vi "Write Log File Directory.vi"(8 "error in (no error)":errorcluster, 10 "Log File Directory":string, 11 "Check Size Message in":refnum<class "Check Size Message.lvclass">) -> (0 "error out":errorcluster, 3 "Check Size Message out":refnum<class "Check Size Message.lvclass">)   [LabVIEW 2020, in "AIM ARINC 664 Engine.lvlib" / "Implementation.lvlib" / "Frame Logging.lvlib" / "Check Size Message.lvclass"]
uses:
  Check Size Message.lvclass
  Check Size Message.lvclass/Check Size Message.ctl
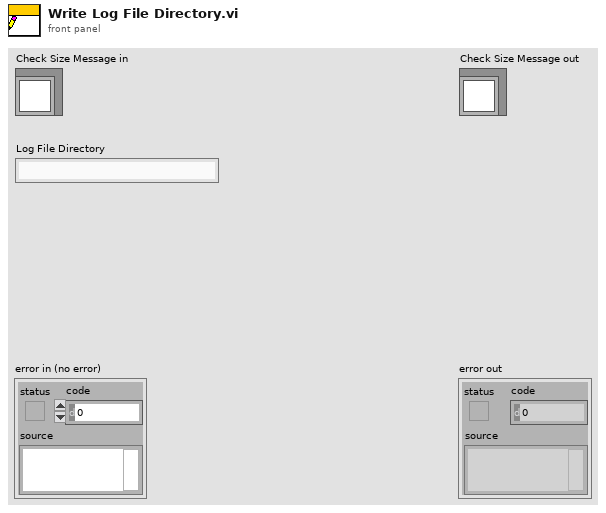
[diagram p1: front panel]
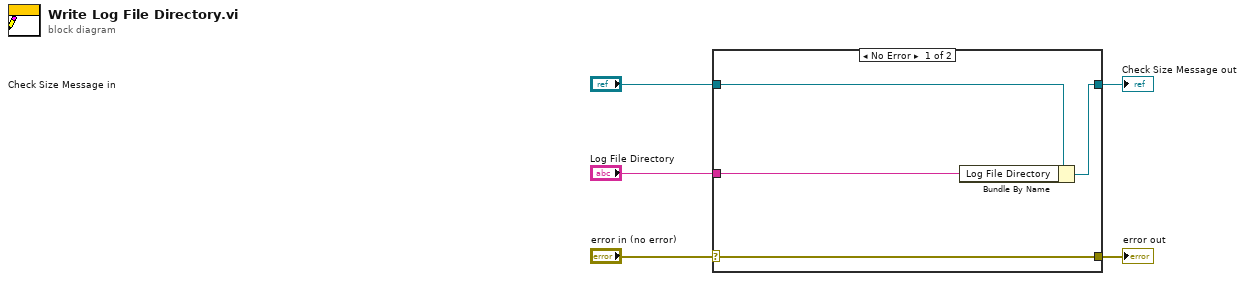
[diagram p0: block diagram]
diagram:
  n1 = case shown="No Error" "error in (no error)" {
    selector: "error in (no error)" -> [w9 w10]
    tunnel: [w9 w10] -> w4
    tunnel: [w7 w11] -> w2
    tunnel: "Check Size Message in" -> [w8 w11]
    tunnel: "Log File Directory" -> [w6 _]
    frame No Error {
      n2 = Bundle By Name(cluster=w8, "Log File Directory"=w6) -> (w7:refnum<class "Check Size Message.lvclass">)
    }
    frame Error {
    }
  }
  "error out" <- w4
  "Check Size Message out" <- w2
